vi "SLSC Remove Channels.vi"(8 "error in (no error)":errorcluster, 11 "Item Ref in":T1 format="%.0x") -> (0 "error out":errorcluster, 3 "Item Ref out":T1 format="%.0x")   [LabVIEW 2015, in "SLSC EDS System Explorer.lvlib"]
uses:
  System Explorer/SLSC EDS System Explorer.lvlib
  <vilib>/NI Veristand/Custom Device API/Custom Device Item Ref.ctl
  <vilib>/NI VeriStand/Custom Device API/Custom Device API.lvlib
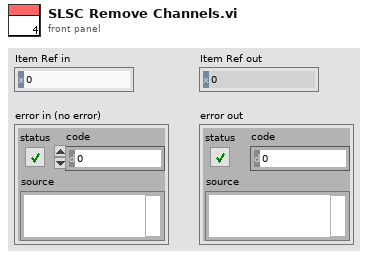
[diagram p1: front panel]
types:
  T1 = typedef "Custom Device API.lvlib/Custom Device Item Ref.ctl" = u64
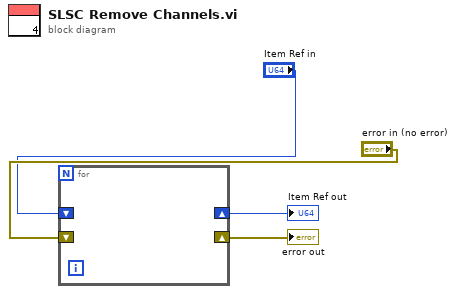
[diagram p0: block diagram]
diagram:
  n1 = for {
    shift-right: [_] -> w2
    shift-left: "Item Ref in" -> [_]
    shift-right: [_] -> w4
    shift-left: "error in (no error)" -> [_]
  }
  "error out" <- w4
  "Item Ref out" <- w2
